vi "Get Size 1D.vi"(8 "error in (no error)":errorcluster, 11 "Abs_Time 1D in":refnum<class "Abs_Time 1D.lvclass">) -> (0 "error out":errorcluster, 2 "Size":i32, 3 "Abs_Time 1D out":refnum<class "Abs_Time 1D.lvclass">)   [LabVIEW 2019, in "Abs_Time 1D.lvclass"]
uses:
  Abs_Time 1D.lvclass
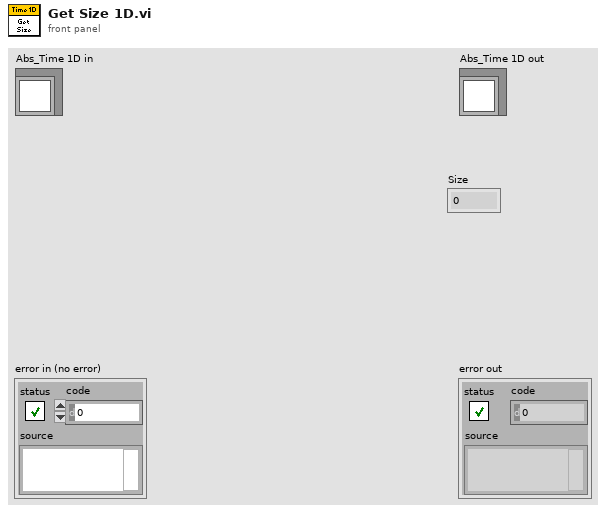
[diagram p1: front panel]
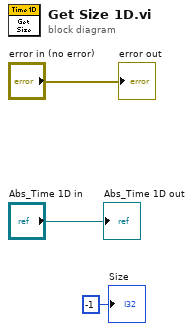
[diagram p0: block diagram]
diagram:
  "error out" <- "error in (no error)"
  "Abs_Time 1D out" <- "Abs_Time 1D in"
  "Size" <- -1 ("Size")
